vi "Get Cell Type.vi"(8 "error in":errorcluster, 10 "Cell in":refnum<k24>, 11 "SpreadsheetDoc in":refnum<k24>) -> (0 "error out":errorcluster, 1 "Type":T1, 2 "Cell out":refnum<k24>, 3 "SpreadsheetDoc out":refnum<k24>)   [LabVIEW 2019, in "Open Xml.lvlib"]
uses:
  Open Xml.lvlib
  D:/git/Open-Xml-LabVIEW/Source/DocumentFormat.OpenXml.dll
  DocumentFormat.OpenXml.dll
  D:/git/Open-Xml-LabVIEW/Source/DocumentFormat.OpenXml.Framework.dll
  DocumentFormat.OpenXml.Framework.dll
  Cell DataType.ctl
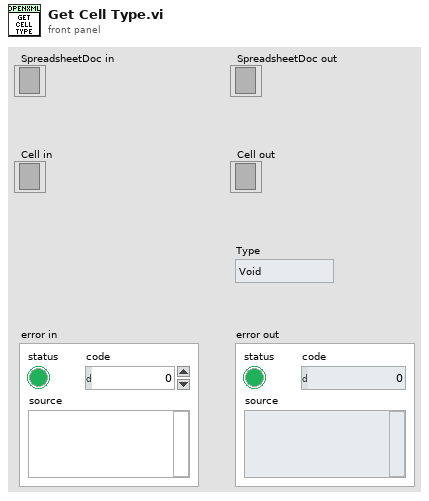
[diagram p1: front panel]
types:
  T1 = typedef "Open Xml.lvlib/Cell DataType.ctl" = enum16{"Void", "Boolean", "Number", "Error", "SharedString", "String", "InlineString", "Date"}
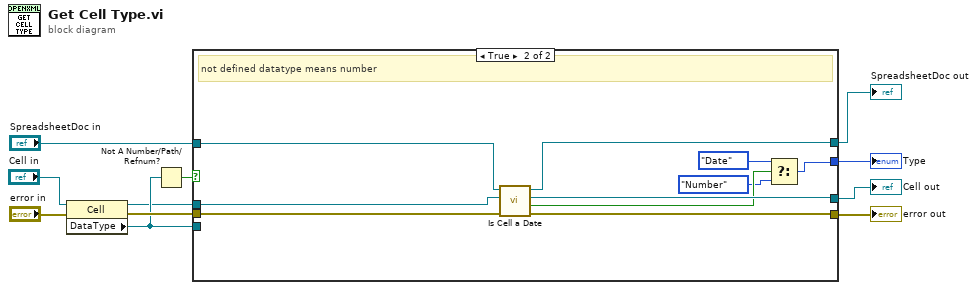
[diagram p0: block diagram]
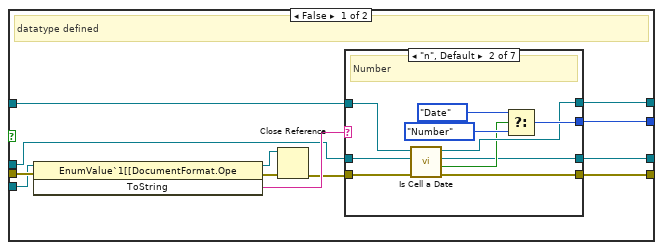
[diagram p2: hidden frame]
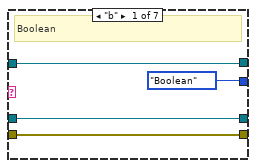
[diagram p3: hidden frame]
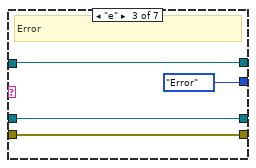
[diagram p4: hidden frame]
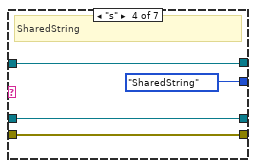
[diagram p5: hidden frame]
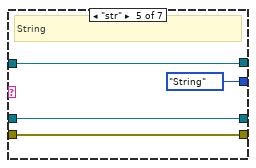
[diagram p6: hidden frame]
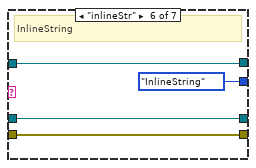
[diagram p7: hidden frame]
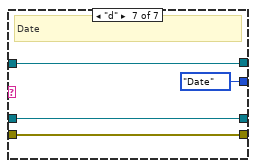
[diagram p8: hidden frame]
diagram:
  n1 = property class="Cell"(reference="Cell in", error in="error in") -> (reference out=w3:refnum<k24>, error out=w9:errorcluster, "DataType"=w4:refnum<k24>)
  n2 = Not A Number/Path/Refnum?(number/path/refnum=w4) -> (NaN/Path/Refnum?=w5:bool)
  n3 = case shown="True" w5 {
    tunnel: [w23 w62] -> w11
    tunnel: w9 -> [w22 w67]
    tunnel: w4 -> [w21 _]
    tunnel: [w17 w65] -> w1
    tunnel: "SpreadsheetDoc in" -> [w20 w64]
    tunnel: [w19 w63] -> w6
    tunnel: [w16 w61] -> w2
    tunnel: w3 -> [w15 w58]
    frame False {
      # "datatype defined"
      n4 = invoke class="EnumValue`1[[DocumentFormat.Ope" method="ToString"(reference=w21, error in=w22) -> (reference out=w14:refnum<k24>, error out=w13:errorcluster, "ToString"=w18:string)  [unwired: 1 in]
      n5 = Close Reference(reference=w14, error in (no error)=w13) -> (error out=w12:errorcluster)
      n6 = case shown="\"n\", Default" w18 {
        tunnel: w12 -> [w27 w36 w40 w43 w49 w53 w57]
        tunnel: [w27 w33 w40 w43 w49 w53 w57] -> w17
        tunnel: [Cell_DataType."Boolean" ("f") w35 Cell_DataType."Error" ("f") Cell_DataType."SharedString" ("f") Cell_DataType."String" ("f") Cell_DataType."InlineString" ("f") Cell_DataType."Date" ("f")] -> w23
        tunnel: w20 -> [w26 w37 w41 w45 w48 w52 w56]
        tunnel: [w26 w34 w41 w45 w48 w52 w56] -> w19
        tunnel: [w24 w29 w38 w42 w46 w50 w54] -> w16
        tunnel: w15 -> [w24 w28 w38 w42 w46 w50 w54]
        frame "b" {
          # "Boolean"
        }
        frame "n", Default {
          # "Number"
          n7 = call "Is Cell a Date.vi"("error in"=w36, "Cell in"=w28, "SpreadsheetDoc in"=w37) -> ("error out"=w33:errorcluster, "Is Date"=w30:bool, "Cell out"=w29:refnum<k24>, "SpreadsheetDoc out"=w34:refnum<k24>)  [unwired: 5 in]
          n8 = Select(t=Cell_DataType."Date" ("enum"), s=w30, f=Cell_DataType."Number") -> (s? t:f=w35:T1)
        }
        frame "e" {
          # "Error"
        }
        frame "s" {
          # "SharedString"
        }
        frame "str" {
          # "String"
        }
        frame "inlineStr" {
          # "InlineString"
        }
        frame "d" {
          # "Date"
        }
      }
    }
    frame True {
      # "not defined datatype means number"
      n9 = call "Is Cell a Date.vi"("error in"=w67, "Cell in"=w58, "SpreadsheetDoc in"=w64) -> ("error out"=w65:errorcluster, "Is Date"=w60:bool, "Cell out"=w61:refnum<k24>, "SpreadsheetDoc out"=w63:refnum<k24>)  [unwired: 5 in]
      n10 = Select(t=Cell_DataType."Date" ("f"), s=w60, f=Cell_DataType."Number") -> (s? t:f=w62:T1)
    }
  }
  "Type" <- w11
  "error out" <- w1
  "Cell out" <- w2
  "SpreadsheetDoc out" <- w6
